vi "RestoreDefaultMDSplusSettings.vi"() -> (0 "Initialized DAQ Array":T4(array[cluster]) {"Card Settings"."Start Time" format="%#_3p"; "Card Settings"."End Time" format="%#_3p"; "Card Settings"."Rate" format="%#_3p"}, 1 "Initialized Timing Array":T5[](array[typedef]) {"Timing Sequence"."Dt" format="%_3p"; "Timing Sequence"."Time" format="%_3p"})   [LabVIEW 2014]
uses:
  Controls/TimingControl.ctl
  Controls/TimingControlChannel.ctl
  Controls/DAQ Card Channel Array.ctl
  Controls/DAQ Channel Settings.ctl
  Controls/DAQ Card Settings.ctl
  Controls/DAQ Card-Channel Settings.ctl
panel:
  # "Sampling Rate [1/s]"
  # "Start Time [s]"
  # "End Time [s]"
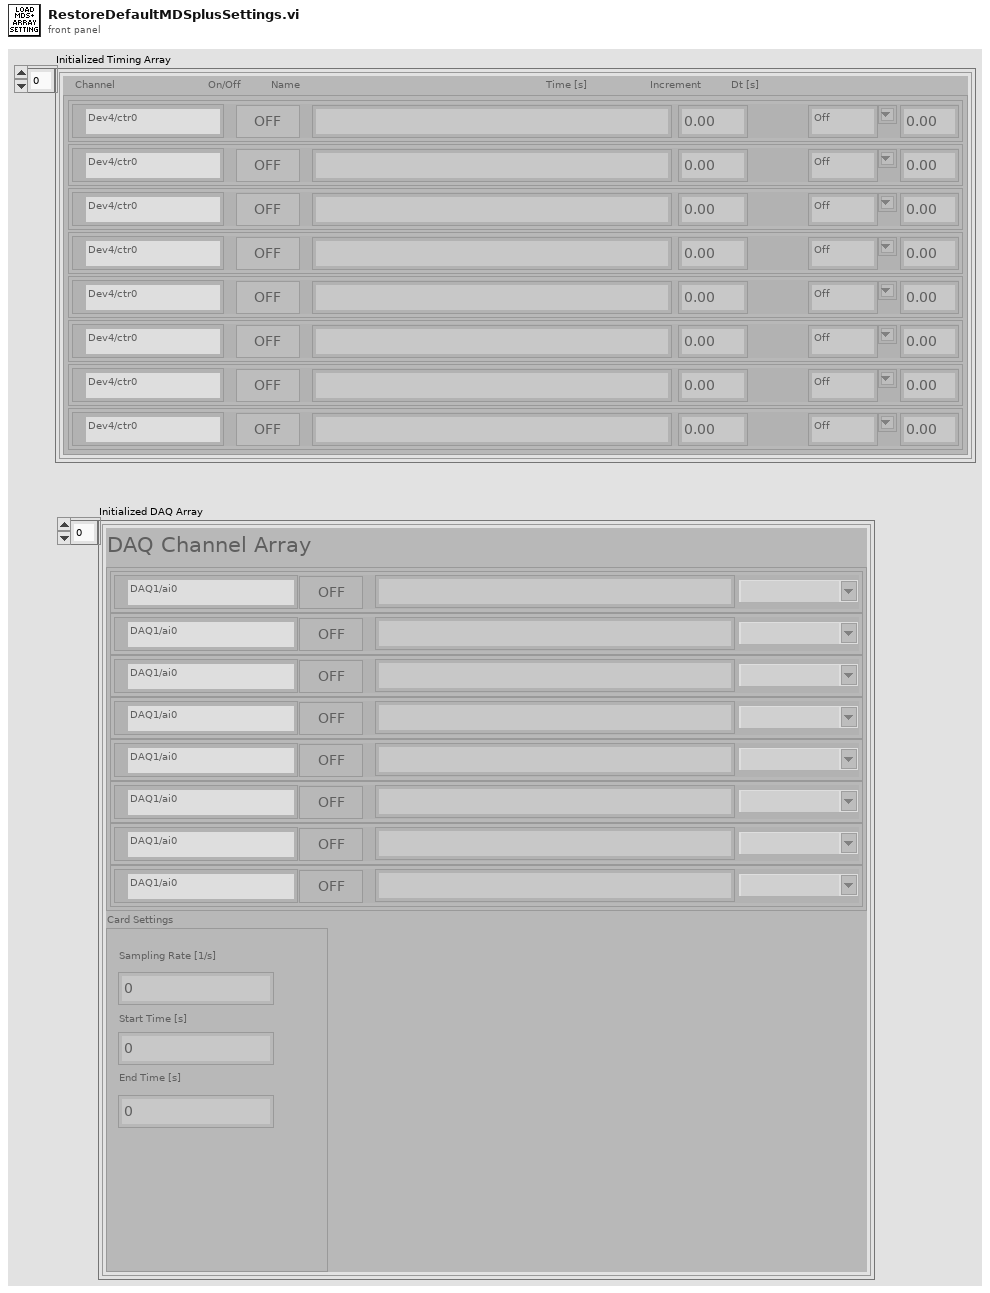
[diagram p1: front panel]
types:
  T1 = typedef "DAQ Card Channel Array.ctl" = T2[]
  T2 = typedef "DAQ Channel Settings.ctl" = cluster{"Active":bool, "Channel Name":string, "Channel":tag, "Voltage Range":string}
  T3 = typedef "DAQ Card Settings.ctl" = cluster{"Rate":dbl, "End Time":dbl, "Start Time":dbl}
  T4 = cluster{"DAQ Channel Array":T1, "Card Settings":T3}[]
  T5 = typedef "TimingControl.ctl" = cluster{"Timing Sequence":T6[]}
  T6 = typedef "TimingControlChannel.ctl" = cluster{"Active":bool, "counter":tag, "Channel Name":string, "Time":dbl, "Increment":string, "Dt":dbl}
  T7 = typedef "DAQ Card-Channel Settings.ctl" = cluster{"DAQ Channel Array":T1, "Card Settings":T3}
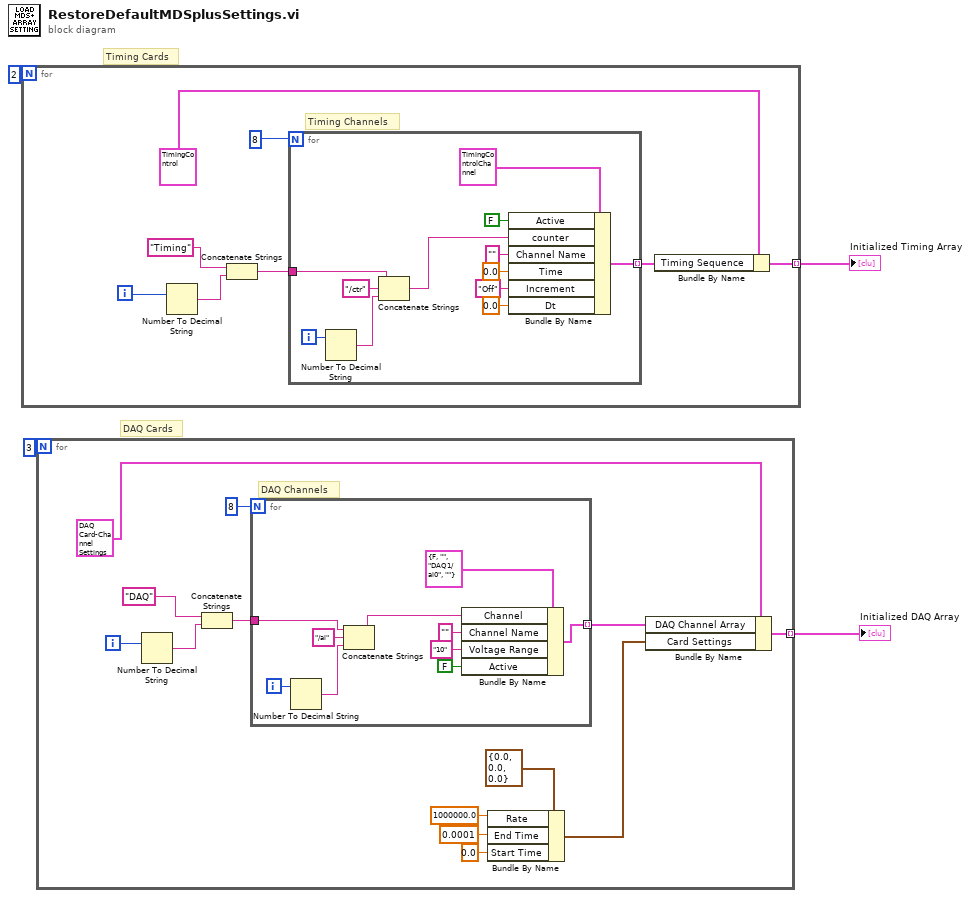
[diagram p0: block diagram]
diagram:
  # "DAQ Cards"
  # "Timing Cards"
  n1 = for {
    N: 2 -> [_]
    tunnel: [w7] -> w3 mode=indexing
    i -> [w8]
    # "Timing Channels"
    n2 = Number To Decimal String(number=w8) -> (decimal integer string=w12:string)  [unwired: 1 in]
    n3 = Concatenate Strings("Timing", w12) -> (w10:string)
    n4 = for {
      N: 8 -> [_]
      tunnel: w10 -> [w23]
      tunnel: [w19] -> w5 mode=indexing
      i -> [w22]
      n5 = Number To Decimal String(number=w22) -> (decimal integer string=w21:string)  [unwired: 1 in]
      n6 = Concatenate Strings(w23, "/ctr" ("string"), w21) -> (w20:string)
      n7 = Bundle By Name(cluster=T6 {"Active"=FALSE, "counter"="PXI1Slot9/ctr7", "Channel Name"="", "Time"=0.0, "Increment"="Off", "Dt"=0.0} ("Counters"), "Active"=FALSE, "counter"=w20, "Channel Name"="", "Time"=0.0, "Increment"="Off", "Dt"=0.0) -> (w19:T6)
    }
    n8 = Bundle By Name(cluster=T5 {"Timing Sequence"=[{"Active"=FALSE, "counter"="PXI1Slot9/ctr7", "Channel Name"="", "Time"=0.0, "Increment"="Off", "Dt"=0.0}, {"Active"=FALSE, "counter"="Dev4/ctr0", "Channel Name"="", "Time"=0.0, "Increment"="Off", "Dt"=0.0}, {"Active"=FALSE, "counter"="Dev4/ctr0", "Channel Name"="", "Time"=0.0, "Increment"="Off", "Dt"=0.0}, {"Active"=FALSE, "counter"="Dev4/ctr0", "Channel Name"="", "Time"=0.0, "Increment"="Off", "Dt"=0.0}, {"Active"=FALSE, "counter"="Dev4/ctr0", "Channel Name"="", "Time"=0.0, "Increment"="Off", "Dt"=0.0}, {"Active"=FALSE, "counter"="Dev4/ctr0", "Channel Name"="", "Time"=0.0, "Increment"="Off", "Dt"=0.0}, {"Active"=FALSE, "counter"="Dev4/ctr0", "Channel Name"="", "Time"=0.0, "Increment"="Off", "Dt"=0.0}, {"Active"=FALSE, "counter"="Dev4/ctr0", "Channel Name"="", "Time"=0.0, "Increment"="Off", "Dt"=0.0}]} ("Cluster"), "Timing Sequence"=w5) -> (w7:T5)
  }
  "Initialized Timing Array" <- w3
  n9 = for {
    N: 3 -> [_]
    tunnel: [w32] -> w1 mode=indexing
    i -> [w37]
    # "DAQ Channels"
    n10 = Number To Decimal String(number=w37) -> (decimal integer string=w36:string)  [unwired: 1 in]
    n11 = Concatenate Strings("DAQ", w36) -> (w34:string)
    n12 = for {
      N: 8 -> [_]
      tunnel: w34 -> [w46]
      tunnel: [w40] -> w30 mode=indexing
      i -> [w45]
      n13 = Number To Decimal String(number=w45) -> (decimal integer string=w44:string)  [unwired: 1 in]
      n14 = Concatenate Strings(w46, "/ai" ("string"), w44) -> (w43:string)
      n15 = Bundle By Name(cluster=T2 {"Active"=FALSE, "Channel Name"="", "Channel"="DAQ1/ai0", "Voltage Range"=""} ("Counters"), "Channel"=w43, "Channel Name"="", "Voltage Range"="10", "Active"=FALSE) -> (w40:T2)
    }
    n16 = Bundle By Name(cluster=T3 {"Rate"=0.0, "End Time"=0.0, "Start Time"=0.0} ("Card Settings"), "Rate"=1000000.0, "End Time"=0.0001, "Start Time"=0.0) -> (w25:T3)
    n17 = Bundle By Name(cluster=T7 {"DAQ Channel Array"=[{"Active"=FALSE, "Channel Name"="", "Channel"="DAQ1/ai0", "Voltage Range"=""}, {"Active"=FALSE, "Channel Name"="", "Channel"="DAQ1/ai0", "Voltage Range"=""}, {"Active"=FALSE, "Channel Name"="", "Channel"="DAQ1/ai0", "Voltage Range"=""}, {"Active"=FALSE, "Channel Name"="", "Channel"="DAQ1/ai0", "Voltage Range"=""}, {"Active"=FALSE, "Channel Name"="", "Channel"="DAQ1/ai0", "Voltage Range"=""}, {"Active"=FALSE, "Channel Name"="", "Channel"="DAQ1/ai0", "Voltage Range"=""}, {"Active"=FALSE, "Channel Name"="", "Channel"="DAQ1/ai0", "Voltage Range"=""}, {"Active"=FALSE, "Channel Name"="", "Channel"="DAQ1/ai0", "Voltage Range"=""}], "Card Settings"={"Rate"=100.0, "End Time"=0.0, "Start Time"=0.0}} ("Cluster"), "DAQ Channel Array"=w30, "Card Settings"=w25) -> (w32:T7)
  }
  "Initialized DAQ Array" <- w1
